vi "PUT X Maximum Extension.vi"(0 "X Maximum Extension":dbl) -> ()   [LabVIEW 2013]
uses:
  Action.ctl
  Physical Constants FGV Selector.ctl
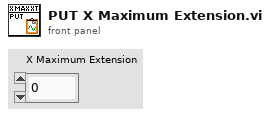
[diagram p1: front panel]
types:
  T1 = typedef "Physical Constants FGV Selector.ctl" = enum16{"Maximum Output Voltage", "Minimum Output Voltage", "Maximum Input Voltage", "Minimum Input Voltage", "X Piezo Response", "X Piezo Max Extension", "X Piezo Min Extension", "Y Piezo Response", "Y Piezo Max Extension", "Y Piezo Min Extension", "Z Piezo Response", "Z Piezo Max Extension", "Z Piezo Min Extension"}
  T2 = typedef "Action.ctl" = enum16{"GET", "PUT", "DELETE"}
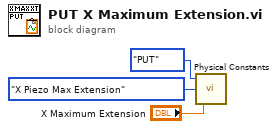
[diagram p0: block diagram]
diagram:
  n1 = call "Physical Constants.vi"("Input"="X Maximum Extension", "Physical Constants FGV Selector"=Physical_Constants_FGV_Selector."X Piezo Max Extension", "Action"=Action."PUT") -> ()  [unwired: 1 out]
